vi "Query Setup.vi"(8 "error in (no error)":errorcluster, 9 "Query Setup File Location":path, 10 "Saved Setup Number (0)":i32, 11 "VISA resource name":refnum<visa-resource-name>) -> (0 "error out":errorcluster, 3 "VISA resource name out":refnum<visa-resource-name>)   [LabVIEW 2014, in "Fluke 190 Series II.lvlib"]
doc: "Queries the ScopeMeter testtool for the present acquisition setup data.\n\n<b>Note:</b>\nYou should specify a path and file to store the queried setup data."
uses:
  Fluke 190 Series II.lvlib
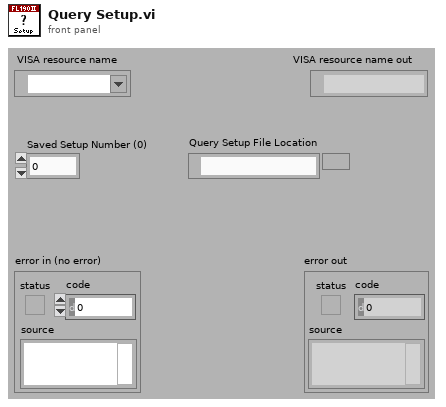
[diagram p1: front panel]
types:
  T1 = enum16{"open", "replace", "create", "open or create", "replace or create", "replace or create with confirmation"}
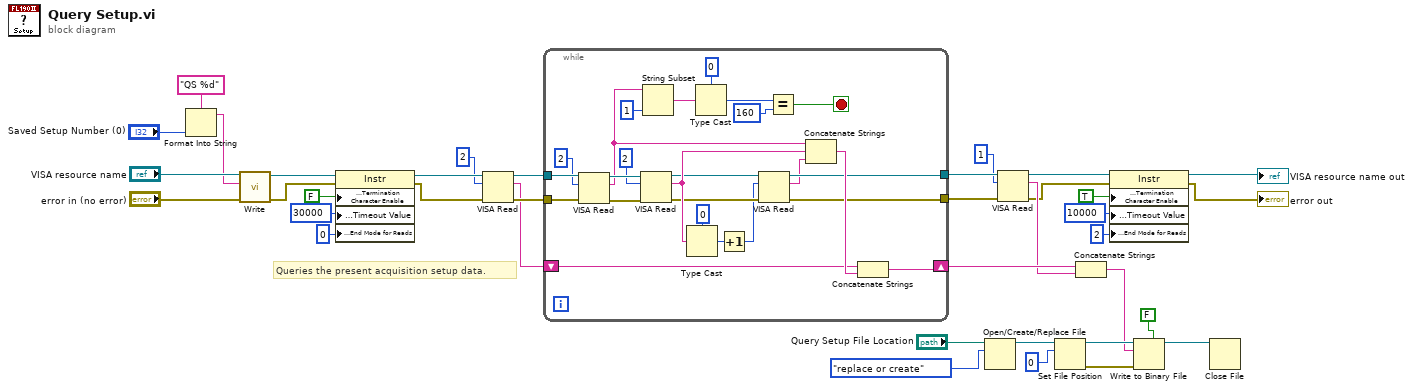
[diagram p0: block diagram]
diagram:
  # "Queries the present acquisition setup data."
  n1 = Format Into String(format string="QS %d", "Saved Setup Number (0)") -> (resulting string=w32:string)  [unwired: 2 in, 1 out]
  n2 = call "Write.vi"("error in (no error)"="error in (no error)", "Write Buffer"=w32, "VISA resource name"="VISA resource name") -> ("error out"=w30:errorcluster, "VISA resource name out"=w31:refnum<visa-resource-name>)  [unwired: 7 out]
  n3 = property class="Instr"(reference=w31, error in=w30, "Message Based Settings:Termination Character Enable"=FALSE, "General Settings:Timeout Value"=u32 30000, "Serial Settings:End Mode for Reads"=u16 0) -> (reference out=w24:refnum<visa-resource-name>, error out=w23:errorcluster)
  n4 = VISA Read(VISA resource name=w24, byte count=u32 2, error in (no error)=w23) -> (VISA resource name out=w26:refnum<visa-resource-name>, read buffer=w10:string, error out=w25:errorcluster)  [unwired: 1 out]
  n5 = while {
    shift-right: [w56] -> w35
    shift-left: w10 -> [w57]
    tunnel: [w43] -> w21
    tunnel: [w42] -> w20
    tunnel: w26 -> [w50]
    tunnel: w25 -> [w51]
    stop <- w61 stop-if-true
    n6 = VISA Read(VISA resource name=w50, byte count=u32 2, error in (no error)=w51) -> (VISA resource name out=w47:refnum<visa-resource-name>, read buffer=w39:string, error out=w48:errorcluster)  [unwired: 1 out]
    n7 = VISA Read(VISA resource name=w47, byte count=u32 2, error in (no error)=w48) -> (VISA resource name out=w44:refnum<visa-resource-name>, read buffer=w46:string, error out=w45:errorcluster)  [unwired: 1 out]
    n8 = String Subset(string=w39, length (rest)=1 ("length (rest)")) -> (substring=w55:string)  [unwired: 1 out]
    n9 = Type Cast(type=u16 0, x=w46) -> (*(type *) &x=w59:u16)
    n10 = Type Cast(type=u8 0, x=w55) -> (*(type *) &x=w53:u8)
    n11 = Increment(x=w59) -> (x+1=w41:u16)
    n12 = VISA Read(VISA resource name=w44, byte count=w41, error in (no error)=w45) -> (VISA resource name out=w43:refnum<visa-resource-name>, read buffer=w38:string, error out=w42:errorcluster)  [unwired: 1 out]
    n13 = Equal?(x=w53, y=u8 160) -> (x = y?=w61:bool)
    n14 = Concatenate Strings(w39, w46, w38) -> (w58:string)
    n15 = Concatenate Strings(w57, w58) -> (w56:string)
  }
  n16 = Open/Create/Replace File(file path (use dialog)="Query Setup File Location", operation (0:open)=T1."replace or create") -> (refnum out=w7:refnum<file>)  [unwired: 4 in, 2 out]
  n17 = VISA Read(VISA resource name=w21, byte count=u32 1, error in (no error)=w20) -> (VISA resource name out=w14:refnum<visa-resource-name>, read buffer=w18:string, error out=w11:errorcluster)  [unwired: 1 out]
  n18 = Set File Position(offset (in bytes) (0)=i64 0, refnum=w7) -> (refnum out=w5:refnum<file>, error out=w4:errorcluster)  [unwired: 1 in, 1 out]
  n19 = Concatenate Strings(w35, w18) -> (w3:string)
  n20 = property class="Instr"(reference=w14, error in=w11, "Message Based Settings:Termination Character Enable"=TRUE, "General Settings:Timeout Value"=u32 10000, "Serial Settings:End Mode for Reads"=u16 2) -> (reference out=→"VISA resource name out":refnum<visa-resource-name>, error out=→"error out":errorcluster)
  n21 = Write to Binary File(file (use dialog)=w5, data=w3, error in=w4, 5:FALSE ("prepend array or string size? (T)")) -> (refnum out=w1:refnum<file>)  [unwired: 4 out]
  n22 = Close File(refnum=w1) -> ()  [unwired: 1 in, 2 out]
